vi "Set Concrete Aggregate.vi"(8 "error in (no error)":errorcluster caption="错误输入（无错误）", 10 "迭代器.lvlib:具体聚集.lvclass":refnum<class "具体聚集.lvclass">, 11 "具体迭代器 输入":refnum<class "具体迭代器.lvclass"> caption="DNL_LabVIEW Object in") -> (0 "error out":errorcluster caption="错误输出", 3 "具体迭代器 输出":refnum<class "具体迭代器.lvclass"> caption="DNL_LabVIEW Object out")   [LabVIEW 2011, in "迭代器.lvlib" / "具体迭代器.lvclass"]
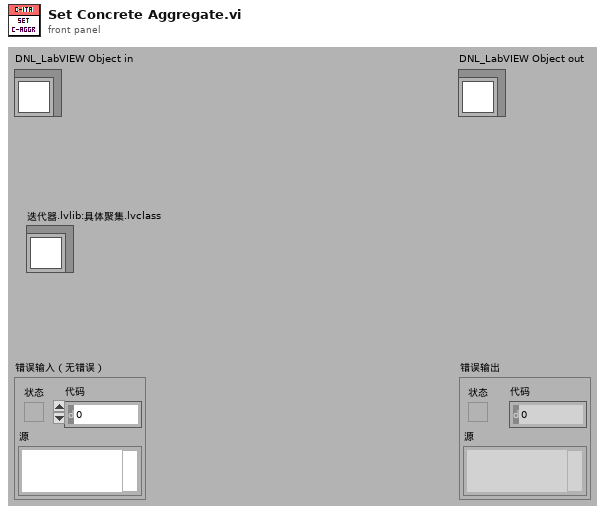
[diagram p1: front panel]
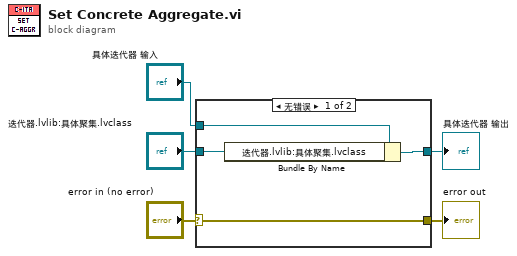
[diagram p0: block diagram]
diagram:
  n1 = case shown="无错误" "error in (no error)" {
    selector: "error in (no error)" -> [w9 w11]
    tunnel: [w9 w11] -> w4
    tunnel: [w7 w10] -> w2
    tunnel: "具体迭代器 输入" -> [w8 w10]
    tunnel: "迭代器.lvlib:具体聚集.lvclass" -> [w6 _]
    frame No Error {
      n2 = Bundle By Name(cluster=w8, "迭代器.lvlib:具体聚集.lvclass"=w6) -> (w7:refnum<class "具体迭代器.lvclass">)
    }
    frame Error {
    }
  }
  "error out" <- w4
  "具体迭代器 输出" <- w2
